vi "min_and_max_array.vi"(8 "error in (no error)":errorcluster, 9 "Maximal amplitute":dbl, 10 "Minimal amplitute":dbl, 11 "Input":dbl[](array[numeric])) -> (0 "error out":errorcluster, 3 "Output":dbl[](array[numeric]))   [LabVIEW 2019]
panel:
  in  "Tab Control":enum32{"Page 1", "Page 2"}(tab)
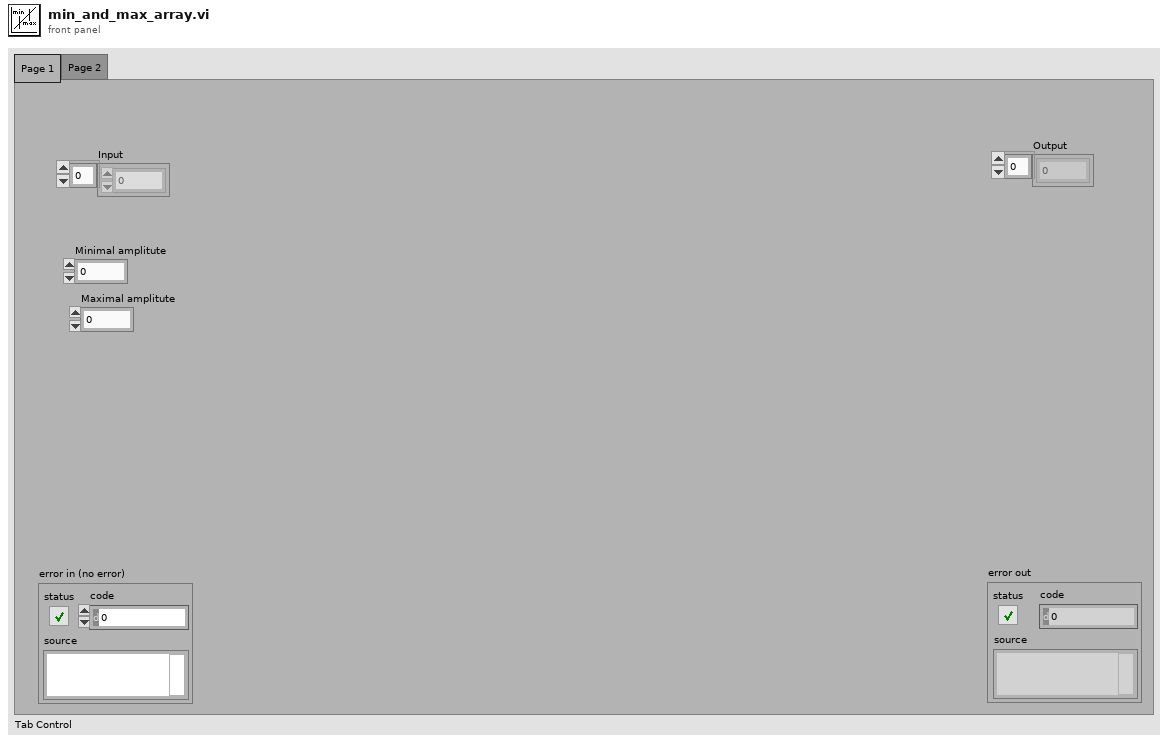
[diagram p1: front panel]
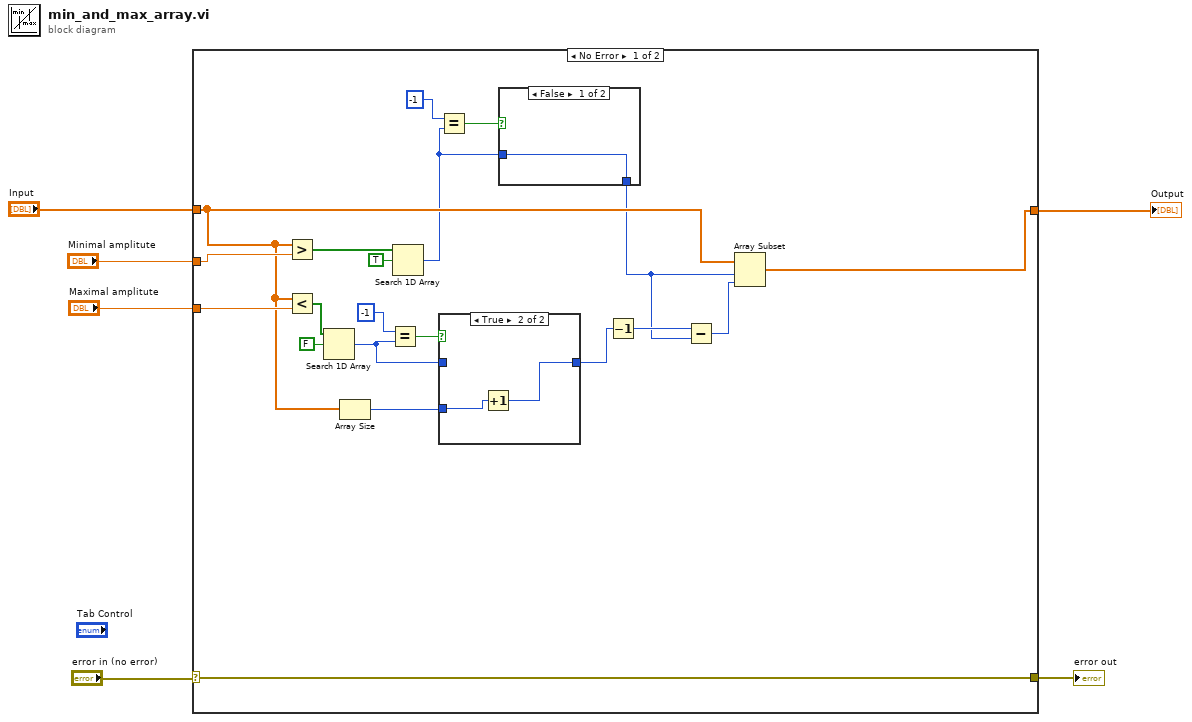
[diagram p0: block diagram]
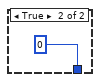
[diagram p2: hidden frame]
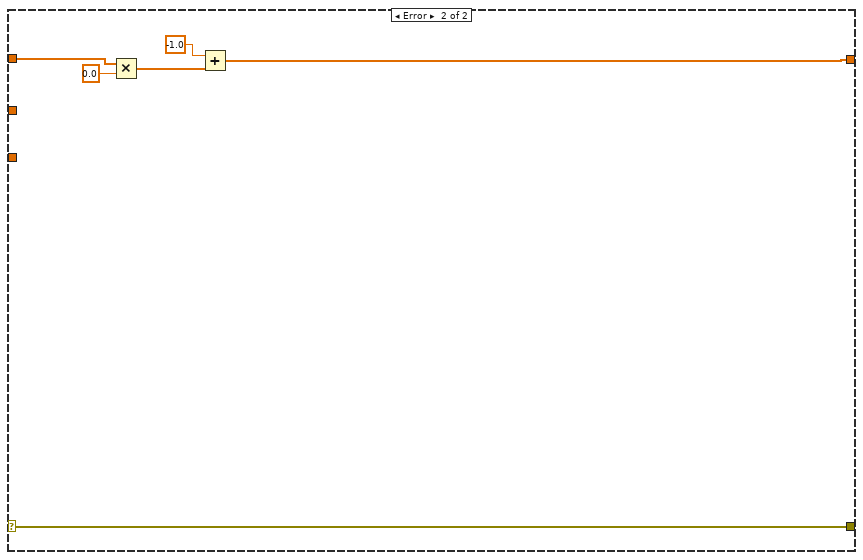
[diagram p4: hidden frame]
diagram:
  n1 = case shown="No Error" "error in (no error)" {
    selector: "error in (no error)" -> [w26 w37]
    tunnel: [w26 w37] -> w5
    tunnel: "Input" -> [w14 w35]
    tunnel: [w18 w32] -> w3
    tunnel: "Minimal amplitute" -> [w25 _]
    tunnel: "Maximal amplitute" -> [w24 _]
    frame No Error {
      n2 = Greater?(x=w14, y=w25) -> (0:w22:bool[])
      n3 = Less?(x=w14, y=w24) -> (x < y?=w23:bool[])
      n4 = Search 1D Array(1D array=w23, element=FALSE) -> (index of element=w11:i32)  [unwired: 1 in]
      n5 = Array Size(array=w14) -> (size(s)=w13:i32)
      n6 = Equal?(x=-1, y=w11) -> (x = y?=w15:bool)
      n7 = Search 1D Array(1D array=w22, element=TRUE) -> (index of element=w7:i32)  [unwired: 1 in]
      n8 = Equal?(x=-1, y=w7) -> (x = y?=w10:bool)
      n9 = case shown="True" w15 {
        tunnel: w13 -> [_ w31]
        tunnel: [w29 w30] -> w12
        tunnel: w11 -> [w29 _]
        frame False {
        }
        frame True {
          n10 = Increment(x=w31) -> (x+1=w30:i32)
        }
      }
      n11 = case shown="False" w10 {
        tunnel: [w27 0] -> w8
        tunnel: w7 -> [w27 _]
        frame False {
        }
        frame True {
        }
      }
      n12 = Decrement(x=w12) -> (x-1=w17:i32)
      n13 = Subtract(x=w17, y=w8) -> (x-y=w19:i32)
      n14 = Array Subset(array=w14, index=w8, length=w19) -> (w18:dbl[])
    }
    frame Error {
      n15 = Multiply(x=w35, y=0.0) -> (x*y=w34:dbl[])
      n16 = Add(x=-1.0 ("y"), y=w34) -> (x+y=w32:dbl[])
    }
  }
  "error out" <- w5
  "Output" <- w3
